vi "Initialize_drivers.vi"(8 "error in (no error)":errorcluster, 11 "Initialize_card in":refnum<class "Control_card.lvclass">) -> (0 "error out":errorcluster, 3 "Initialize_card out":refnum<class "Control_card.lvclass">)   [LabVIEW 2015, in "Control_card.lvclass"]
uses:
  Control_card.lvclass
panel:
  out "System Count":i32
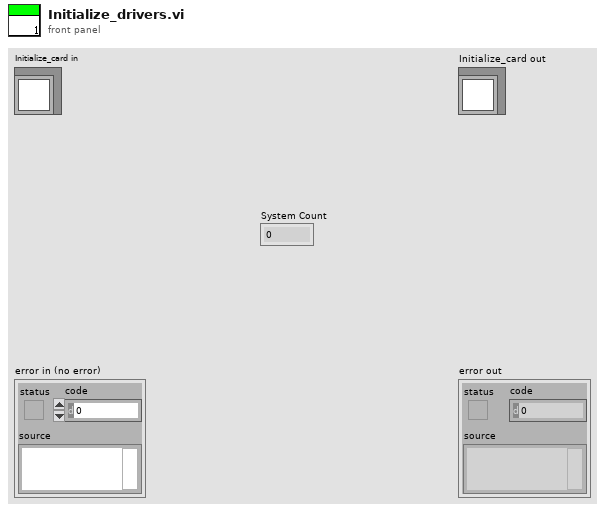
[diagram p1: front panel]
types:
  T1 = cluster{"Handle":u32, "Sample size":u32, "Resolution":i32, "Offset":i32, "Channels":u32, "Boards":u32}
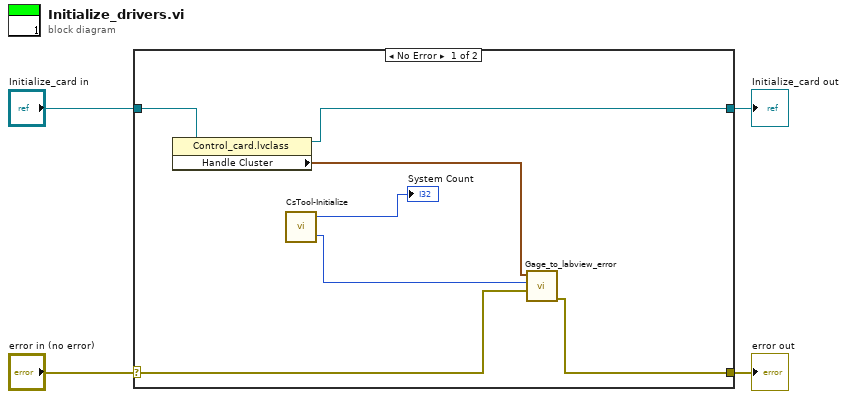
[diagram p0: block diagram]
diagram:
  n1 = case shown="No Error" "error in (no error)" {
    selector: "error in (no error)" -> [w6 w13]
    tunnel: [w5 w13] -> w3
    tunnel: [w8 w12] -> w1
    tunnel: "Initialize_card in" -> [w9 w12]
    frame No Error {
      n2 = property class="Control_card.lvclass"(reference=w9) -> (reference out=w8:refnum<class "Control_card.lvclass">, "Handle Cluster"=w7:T1)  [unwired: 1 in, 1 out]
      n3 = call <userlib>:"CsTool-Initialize.vi"() -> ("Error Code"=w10:i32, "Number Of Systems"=→"System Count":i32)
      n4 = call "Gage_to_labview_error.vi"("Error In"=w6, "GaGe Error Number"=w10, "Handle Cluster"=w7) -> ("Error Out"=w5:errorcluster)  [unwired: 8 in]
    }
    frame Error {
    }
  }
  "error out" <- w3
  "Initialize_card out" <- w1
